vi "Search for Linked List.vi"(7 "Linked List ID":string, 8 "error in (no error)":errorcluster, 10 "Name":string, 11 "Linked List in":refnum<class "Linked List.lvclass">) -> (0 "error out":errorcluster, 2 "IDs":string[](array[string]), 3 "Linked List out":refnum<class "Linked List.lvclass">)   [LabVIEW 2020, in "Linked Lists.lvlib" / "Linked List.lvclass"]
uses:
  <vilib>/gpm_packages/@cs/linked-list/Source/Linked List/Linked List/Linked List.lvclass
  <vilib>/gpm_packages/@cs/linked-list/Source/Linked List/Linked List Definition/Linked List Definition.lvclass
  <vilib>/gpm_packages/@cs/linked-list/Source/Linked List/Linked List/Linked List.lvclass/Linked List.ctl
  <vilib>/gpm_packages/@cs/lookup-table/Source/LookupTable/LookupTable.lvclass/LookupTable.ctl
  3d7f4a9a-e650-4d06-8acf-6c8a7b50f671.vi
  bfa7923c-1809-48cd-8df4-e2ace631b87c.vi
  <vilib>/gpm_packages/@cs/lookup-table/Source/LookupTable/Read Table Reference.vi
  3d7f4a9a-e650-4d06-8acf-6c8a7b50f671.vi/5a7267ad-595e-4610-9ac2-8bef780848ff.vi
  bfa7923c-1809-48cd-8df4-e2ace631b87c.vi/5a7267ad-595e-4610-9ac2-8bef780848ff.vi
  <vilib>/gpm_packages/@cs/lookup-table/Source/LookupTable/LookupTable.lvclass
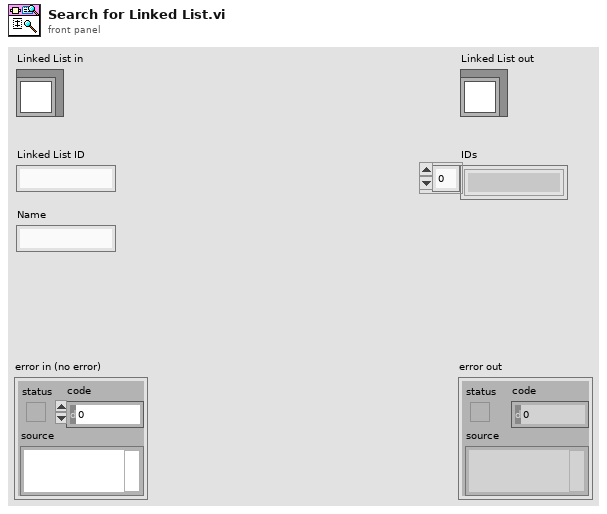
[diagram p1: front panel]
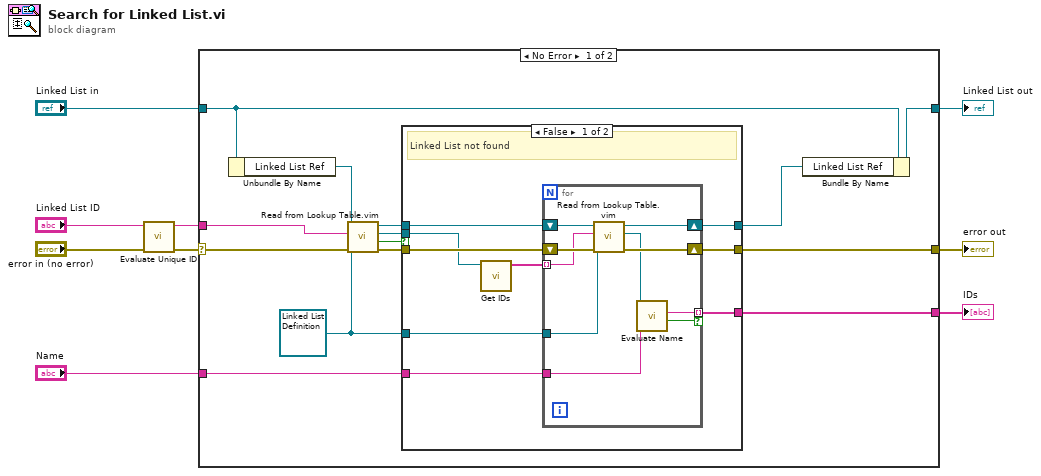
[diagram p0: block diagram]
diagram:
  n1 = call <vilib>:"Evaluate Unique ID.vi"("error in (no error)"="error in (no error)", "Unique ID"="Linked List ID") -> ("error out"=w7:errorcluster, "Unique ID Out"=w6:string)  [unwired: 8 in]
  n2 = case shown="No Error" w7 {
    selector: w7 -> [w23 w46]
    tunnel: w6 -> [w21 _]
    tunnel: "Name" -> [w16 _]
    tunnel: "Linked List in" -> [w15 w45]
    tunnel: [w14 w45] -> w3
    tunnel: [w12 w46] -> w2
    tunnel: [w11 _] -> w1
    frame No Error {
      w18 = refnum<class "Linked List Definition.lvclass"> refnum ("Linked List.lvlib:Linked List Definition.lvclass")
      n3 = Unbundle By Name(w15) -> ("Linked List Ref"=w22:refnum<data-value>)
      n4 = call "Read from Lookup Table.vim"("error in (no error)"=w23, "Type"=w18, "Item Name"=w21, "LookupTable Reference"=w22) -> ("error out"=w20:errorcluster, "Not Found?"=w10:bool, "Value"=w17:refnum<class "Linked List Definition.lvclass">, "LookupTable Reference Out"=w19:refnum<data-value>)  [unwired: 4 in]
      n5 = case shown="False" w10 {
        tunnel: w20 -> [w32 w43]
        tunnel: w19 -> [w31 w44]
        tunnel: w18 -> [w29 _]
        tunnel: w17 -> [w28 _]
        tunnel: w16 -> [w27 _]
        tunnel: [w26 w44] -> w13
        tunnel: [w25 w43] -> w12
        tunnel: [w24 _] -> w11
        frame False {
          # "Linked List not found"
          n6 = call <vilib>:"Get IDs.vi"("Linked List Definition in"=w28) -> ("Child IDs"=w30:string[])  [unwired: 8 in, 2 out]
          n7 = for {
            shift-right: [w40] -> w26
            shift-left: w31 -> [w42]
            shift-right: [w39] -> w25
            shift-left: w32 -> [w41]
            tunnel: w30 -> [w37] mode=indexing
            tunnel: w29 -> [w38]
            tunnel: w27 -> [w35]
            tunnel: [w34] -> w24 mode=indexing if=w33
            n8 = call "Read from Lookup Table.vim"("error in (no error)"=w41, "Type"=w38, "Item Name"=w37, "LookupTable Reference"=w42) -> ("error out"=w39:errorcluster, "Value"=w36:refnum<class "Linked List Definition.lvclass">, "LookupTable Reference Out"=w40:refnum<data-value>)  [unwired: 4 in, 1 out]
            n9 = call <vilib>:"Evaluate Name.vi"("Name"=w35, "Linked List Definition in"=w36) -> ("Match"=w33:bool, "Unique ID"=w34:string)  [unwired: 7 in, 1 out]
          }
        }
        frame True {
          # "Linked List found"
        }
      }
      n10 = Bundle By Name(cluster=w15, "Linked List Ref"=w13) -> (w14:refnum<class "Linked List.lvclass">)
    }
    frame Error {
    }
  }
  "error out" <- w2
  "Linked List out" <- w3
  "IDs" <- w1
